vi "Diff Terminals and Frames.vi"(5 "port old":T2, 7 "port new":T2, 10 "change type":T1, 11 "refresh items in":T11[](array[typedef])) -> (3 "refresh items out":T11[](array[typedef]))   [LabVIEW 2020, in "AIM MIL-STD-1553 System Explorer.lvlib" / "Implementation.lvlib" / "Refresh.lvlib"]
uses:
  Refresh.lvlib
  MCL Row.ctl
  Change Type.ctl
  Symbols.ctl
  Shared/BIU Configuration.ctl
  Shared/Address.ctl
  Shared/Major Frame Definition.ctl
  Shared/Minor Frame Definition.ctl
  Shared/Acyclic Frame Definition.ctl
  Shared/Message Definition.ctl
  Shared/Message Type.ctl
  Shared/Terminal Endpoint.ctl
  Shared/Parameter Definition.ctl
  Name to Symbol.vi
  Scripting/Constants.vi
  Scripting/AIM MIL-STD-1553 Scripting.lvlib
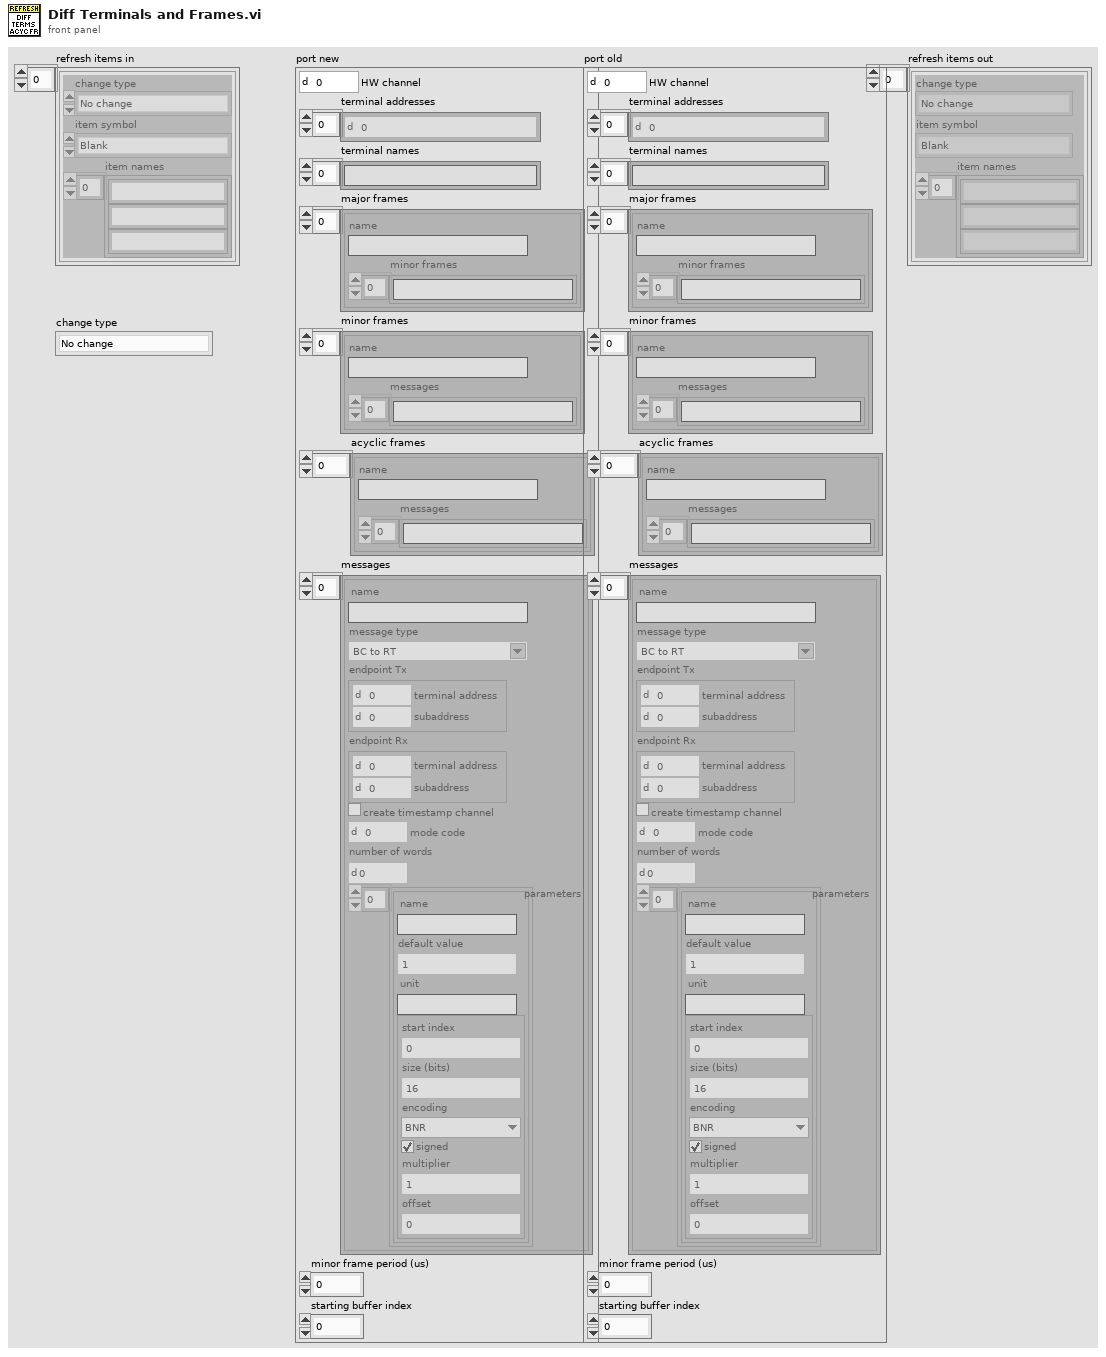
[diagram p1: front panel]
types:
  T1 = typedef "AIM MIL-STD-1553 System Explorer.lvlib/Implementation.lvlib/Refresh.lvlib/Change Type.ctl" = enum16{"No change", "Modify", "Add", "Remove"}
  T2 = typedef "BIU Configuration.ctl" = cluster{"HW channel":u16, "terminal addresses":T3[], "terminal names":string[], "major frames":T4[], "minor frames":T5[], "acyclic frames":T6[], "messages":T7[], "minor frame period (us)":i32, "starting buffer index":u16}
  T3 = typedef "Address.ctl" = u16
  T4 = typedef "Major Frame Definition.ctl" = cluster{"name":string, "minor frames":string[]}
  T5 = typedef "Minor Frame Definition.ctl" = cluster{"name":string, "messages":string[]}
  T6 = typedef "Acyclic Frame Definition.ctl" = cluster{"name":string, "messages":string[]}
  T7 = typedef "Message Definition.ctl" = cluster{"name":string, "message type":T8, "endpoint Tx":T9, "endpoint Rx":T9, "create timestamp channel":bool, "mode code":u16, "number of words":u16, "parameters":cluster{"name":string, "default value":dbl, "unit":string, "parameter definition":T10}[]}
  T8 = typedef "Message Type.ctl" = string
  T9 = typedef "Terminal Endpoint.ctl" = cluster{"terminal address":T3, "subaddress":T3}
  T10 = typedef "Parameter Definition.ctl" = cluster{"start index":i32, "size (bits)":i32, "encoding":enum16{"BNR", "BCD", "Discrete"}, "signed":bool, "multiplier":dbl, "offset":dbl}
  T11 = typedef "AIM MIL-STD-1553 System Explorer.lvlib/Implementation.lvlib/Refresh.lvlib/MCL Row.ctl" = cluster{"change type":T1, "item symbol":T12, "item names":string[]}
  T12 = typedef "AIM MIL-STD-1553 System Explorer.lvlib/Implementation.lvlib/Refresh.lvlib/Symbols.ctl" = enum16{"Blank", "MIL-STD-1553", "Port", "Remote Terminal", "Subaddress", "Bus Controller", "Frame", "Mode Code", "Message", "Parameter", "Item"}
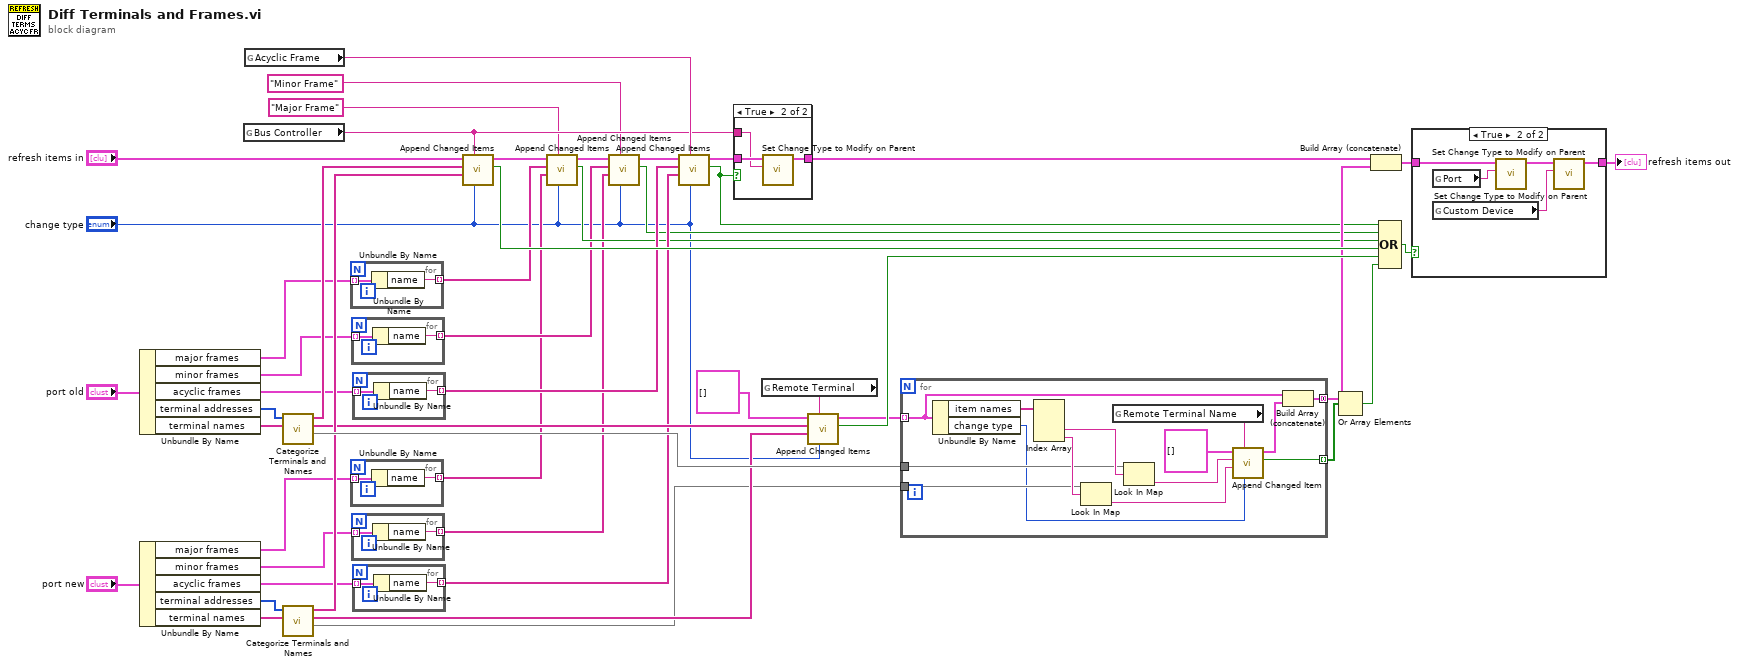
[diagram p0: block diagram]
diagram:
  n1 = Unbundle By Name("port old") -> ("major frames"=w14:T4[], "minor frames"=w15:T5[], "acyclic frames"=w21:T6[], "terminal addresses"=w39:T3[], "terminal names"=w37:string[])
  n2 = Unbundle By Name("port new") -> ("major frames"=w16:T4[], "minor frames"=w17:T5[], "acyclic frames"=w19:T6[], "terminal addresses"=w29:T3[], "terminal names"=w28:string[])
  n3 = global read "Constants.vi" "Bus Controller"() -> (w42:string)
  n4 = global read "Constants.vi" "Acyclic Frame"() -> (w49:string)
  n5 = call "Categorize Terminals and Names.vi"("terminal names"=w37, "terminal addresses"=w39) -> ("map from terminal address (string) to terminal name"=w32:map{string, string}, "remote terminals"=w22:string[], "bus controller"=w47:string[])  [unwired: 7 in]
  n6 = call "Categorize Terminals and Names.vi"("terminal names"=w28, "terminal addresses"=w29) -> ("map from terminal address (string) to terminal name"=w25:map{string, string}, "remote terminals"=w26:string[], "bus controller"=w27:string[])  [unwired: 7 in]
  n7 = for {
    tunnel: [w50] -> _ mode=indexing
    tunnel: [w51] -> w7 mode=indexing
    tunnel: w14 -> [w50] mode=indexing
    n8 = Unbundle By Name(w50) -> ("name"=w51:string)
  }
  n9 = for {
    tunnel: [w52] -> _ mode=indexing
    tunnel: [w53] -> w5 mode=indexing
    tunnel: w16 -> [w52] mode=indexing
    n10 = Unbundle By Name(w52) -> ("name"=w53:string)
  }
  n11 = for {
    tunnel: [w54] -> _ mode=indexing
    tunnel: [w55] -> w6 mode=indexing
    tunnel: w15 -> [w54] mode=indexing
    n12 = Unbundle By Name(w54) -> ("name"=w55:string)
  }
  n13 = for {
    tunnel: w17 -> [w57] mode=indexing
    tunnel: [w56] -> w4 mode=indexing
    n14 = Unbundle By Name(w57) -> ("name"=w56:string)
  }
  n15 = for {
    tunnel: w21 -> [w59] mode=indexing
    tunnel: [w58] -> w20 mode=indexing
    n16 = Unbundle By Name(w59) -> ("name"=w58:string)
  }
  n17 = for {
    tunnel: w19 -> [w61] mode=indexing
    tunnel: [w60] -> w18 mode=indexing
    n18 = Unbundle By Name(w61) -> ("name"=w60:string)
  }
  n19 = call "Append Changed Items.vi"("change type"="change type", "item name"=w42, "items new"=w27, "items old"=w47, "refresh items in"="refresh items in") -> ("modify parent"=w44:bool, "refresh items out"=w13:T11[])  [unwired: 5 in]
  n20 = call "Append Changed Items.vi"("change type"="change type", "item name"="Major Frame", "items new"=w5, "items old"=w7, "refresh items in"=w13) -> ("modify parent"=w8:bool, "refresh items out"=w12:T11[])  [unwired: 5 in]
  n21 = call "Append Changed Items.vi"("change type"="change type", "item name"="Minor Frame", "items new"=w4, "items old"=w6, "refresh items in"=w12) -> ("modify parent"=w9:bool, "refresh items out"=w11:T11[])  [unwired: 5 in]
  n22 = call "Append Changed Items.vi"("change type"="change type", "item name"=w49, "items new"=w18, "items old"=w20, "refresh items in"=w11) -> ("modify parent"=w10:bool, "refresh items out"=w45:T11[])  [unwired: 5 in]
  n23 = case shown="True" w10 {
    tunnel: w45 -> [w62 w65]
    tunnel: [w62 w64] -> w36
    tunnel: w42 -> [_ w63]
    frame False {
    }
    frame True {
      n24 = call "Set Change Type to Modify on Parent.vi"("parent name"=w63, "refresh items in"=w65) -> ("refresh items out"=w64:T11[])  [unwired: 9 in]
    }
  }
  n25 = global read "Constants.vi" "Remote Terminal"() -> (w48:string)
  n26 = call "Append Changed Items.vi"("change type"="change type", "item name"=w48, "items new"=w26, "items old"=w22, "refresh items in"=T11[] []) -> ("modify parent"=w34:bool, "refresh items out"=w33:T11[])  [unwired: 5 in]
  n27 = for {
    tunnel: w33 -> [w72] mode=indexing
    tunnel: w32 -> [w76]
    tunnel: w25 -> [w75]
    tunnel: [w70] -> w31 mode=indexing
    tunnel: [w69] -> w23 mode=concatenating
    n28 = Unbundle By Name(w72) -> ("item names"=w79:string[], "change type"=w73:T1)
    n29 = Index Array(array=w79) -> (element #2=w78:string, element #3=w77:string)  [unwired: 3 in, 1 out]
    n30 = Look In Map(map=w75, key=w77) -> (value=w67:string)  [unwired: 1 in, 1 out]
    n31 = global read "Constants.vi" "Remote Terminal Name"() -> (w66:string)
    n32 = Look In Map(map=w76, key=w78) -> (value=w74:string)  [unwired: 1 in, 1 out]
    n33 = call "Append Changed Item.vi"("change type"=w73, "item name"=w66, "new value"=w67, "old value"=w74, "refresh items in"=T11[] []) -> ("modify parent"=w70:bool, "refresh items out"=w71:T11[])  [unwired: 5 in]
    n34 = Build Array (concatenate)(w72, w71) -> (w69:T11[])
  }
  n35 = Or Array Elements(Boolean array=w31) -> (logical OR=w24:bool)
  n36 = Build Array (concatenate)(w36, w23) -> (w35:T11[])
  n37 = Compound Arithmetic op=OR(w10, w9, w8, w44, w34, w24) -> (w43:bool)
  n38 = case shown="True" w43 {
    tunnel: w35 -> [w80 w85]
    tunnel: [w80 w82] -> w41
    frame False {
    }
    frame True {
      n39 = global read "Constants.vi" "Port"() -> (w84:string)
      n40 = global read "Constants.vi" "Custom Device"() -> (w81:string)
      n41 = call "Set Change Type to Modify on Parent.vi"("parent name"=w84, "refresh items in"=w85) -> ("refresh items out"=w83:T11[])  [unwired: 9 in]
      n42 = call "Set Change Type to Modify on Parent.vi"("parent name"=w81, "refresh items in"=w83) -> ("refresh items out"=w82:T11[])  [unwired: 9 in]
    }
  }
  "refresh items out" <- w41
